vi "change all descriptions.vi"(6 "Prompt?":bool, 9 "new":string, 10 "Path":path, 11 "dataset in":string[][](array[string])) -> (2 "adjust all":bool, 3 "dataset out":string[][](array[string]))   [LabVIEW 2013, in "update vi properties.lvlib"]
uses:
  update vi properties.lvlib
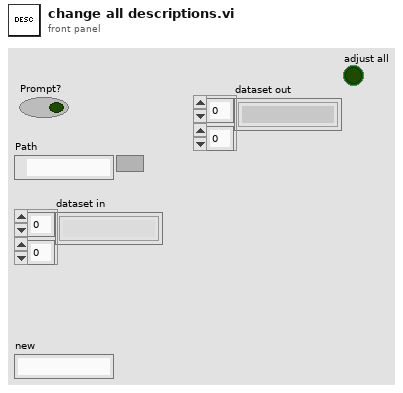
[diagram p1: front panel]
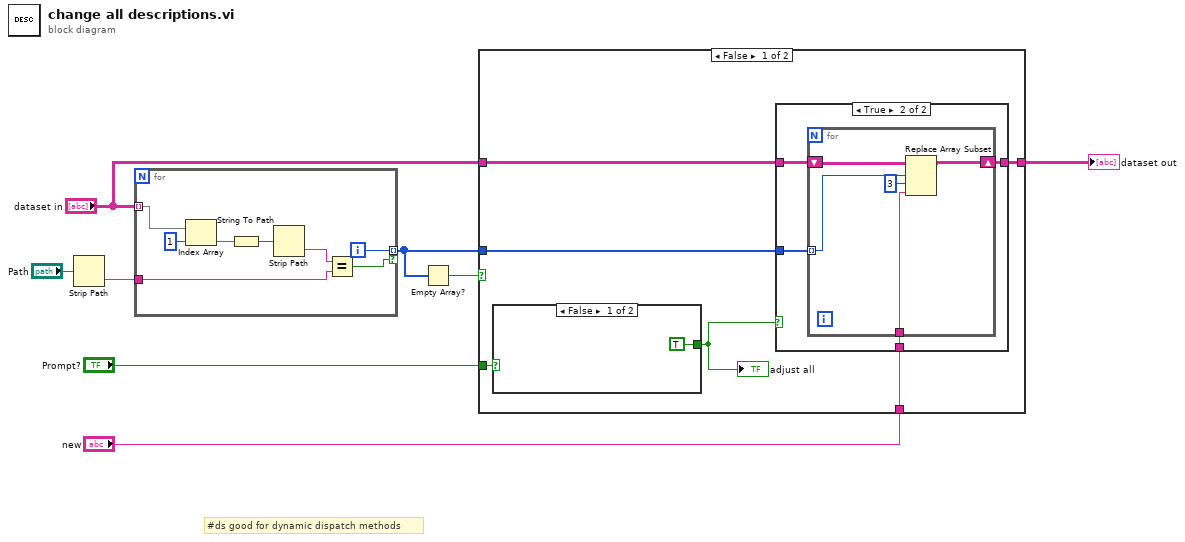
[diagram p0: block diagram]
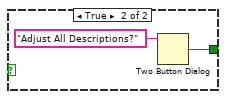
[diagram p2: hidden frame]
diagram:
  # "#ds good for dynamic dispatch methods"
  n1 = Strip Path(path="Path") -> (name=w7:string)  [unwired: 1 out]
  n2 = for {
    tunnel: "dataset in" -> [w11] mode=indexing
    tunnel: w7 -> [w13]
    tunnel: [w10] -> w3 mode=indexing if=w9
    i -> [w10]
    n3 = Index Array(array=w11, index=1) -> (element=w15:string)
    n4 = String To Path(string=w15) -> (path=w14:path)
    n5 = Strip Path(path=w14) -> (name=w12:string)  [unwired: 1 out]
    n6 = Equal?(x=w12, y=w13) -> (x = y?=w9:bool)
  }
  n7 = Empty Array?(array=w3) -> (empty?=w5:bool)
  n8 = case shown="False" w5 {
    tunnel: "dataset in" -> [w21 w36]
    tunnel: [w20 w36] -> w4
    tunnel: w3 -> [w22 _]
    tunnel: "Prompt?" -> [w19 _]
    tunnel: "new" -> [w17 _]
    frame False {
      n9 = case shown="False" w19 {
        tunnel: [TRUE ("T button?") w24] -> w18
        frame False {
        }
        frame True {
          n10 = Two Button Dialog(message="Adjust All Descriptions?") -> (T button?=w24:bool)  [unwired: 2 in]
        }
      }
      "adjust all" <- w18
      n11 = case shown="True" w18 {
        tunnel: w22 -> [_ w30]
        tunnel: w21 -> [w26 w29]
        tunnel: [w26 w28] -> w20
        tunnel: w17 -> [_ w27]
        frame False {
        }
        frame True {
          n12 = for {
            tunnel: w30 -> [w33] mode=indexing
            shift-right: [w34] -> w28
            shift-left: w29 -> [w35]
            tunnel: w27 -> [w31]
            n13 = Replace Array Subset(array=w35, new element=w31, index (row)=w33, index (col)=3 ("disabled index (col)")) -> (w34:string[][])
          }
        }
      }
    }
    frame True {
    }
  }
  "dataset out" <- w4
